vi "tcs_getNextSample_kernelPointingModel.vi"(8 "error in (no error)":errorcluster, 11 "kernel_PointingModel_Ctl":T1={"Coeffv[100]"=[0.0, 0.0, 0.0, 0.0, 0.0, 0.0, 0.0, 0.0, 0.0, 0.0, 0.0, 0.0, 0.0, 0.0, 0.0, 0.0, 0.0, 0.0, 0.0, 0.0, 0.0, 0.0, 0.0, 0.0, 0.0, 0.0, 0.0, 0.0, 0.0, 0.0, 0.0, 0.0, 0.0, 0.0, 0.0, 0.0, 0.0, 0.0, 0.0, 0.0, 0.0, 0.0, 0.0, 0.0, 0.0, 0.0, 0.0, 0.0, 0.0, 0.0, 0.0, 0.0, 0.0, 0.0, 0.0, 0.0, 0.0, 0.0, 0.0, 0.0, 0.0, 0.0, 0.0, 0.0, 0.0, 0.0, 0.0, 0.0, 0.0, 0.0, 0.0, 0.0, 0.0, 0.0, 0.0, 0.0, 0.0, 0.0, 0.0, 0.0, 0.0, 0.0, 0.0, 0.0, 0.0, 0.0, 0.0, 0.0, 0.0, 0.0, 0.0, 0.0, 0.0, 0.0, 0.0, 0.0, 0.0, 0.0, 0.0, 0.0], "Model[30]"=[0, 0, 0, 0, 0, 0, 0, 0, 0, 0, 0, 0, 0, 0, 0, 0, 0, 0, 0, 0, 0, 0, 0, 0, 0, 0, 0, 0, 0, 0], "Nterml"=0, "Nterms"=0, "Ntermx"=0}) -> (0 "error out":errorcluster, 2 "function return":i32, 3 "kernel_PointingModel_Ctl out":T1)   [LabVIEW 2016, in "SALLV_tcs.lvlib"]
doc: "int tcs_shm_getNextSample_kernel_PointingModelLV(tcs_kernel_PointingModelLV *kernel_PointingModel_Ctl );"
uses:
  SALLV_tcs.lvlib
  DataTypes/kernel_PointingModel.ctl
  SALLV_tcs.so
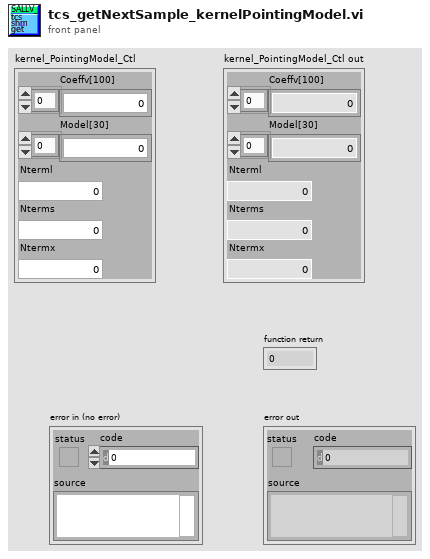
[diagram p1: front panel]
types:
  T1 = typedef "SALLV_tcs.lvlib/kernel_PointingModel.ctl" = cluster{"Coeffv[100]":sgl[], "Model[30]":i32[], "Nterml":i32, "Nterms":i32, "Ntermx":i32}
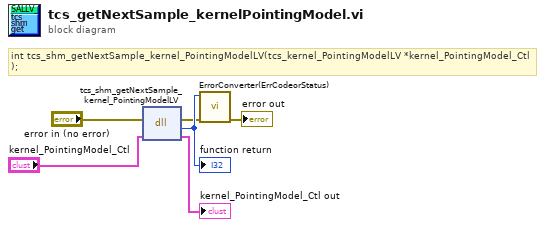
[diagram p0: block diagram]
diagram:
  # "int tcs_shm_getNextSample_kernel_PointingModelLV(tcs_kernel_PointingModelLV *kernel_PointingModel_Ctl );"
  n1 = dll-call lib="home/andres/Desktop/SALLV_tcs/SALLV_tcs.*" fn="tcs_shm_getNextSample_kernel_PointingModelLV"(error in="error in (no error)", "kernel_PointingModel_Ctl"="kernel_PointingModel_Ctl") -> (error out=w2:errorcluster, w6:i32, "kernel_PointingModel_Ctl"=→"kernel_PointingModel_Ctl out":T1)  [unwired: 2 in, 1 out]
  "function return" <- w6
  n2 = call "ErrorConverter(ErrCodeorStatus).vi"("error in (no error)"=w2, "error code"=w6) -> ("error out"=→"error out":errorcluster)  [unwired: 9 in]
